vi "tpg361_ERR.vi"() -> ()   [LabVIEW 2019]
panel:
  out "Error Status":string
  out "Overall Status":bool
  out "Acknowledgement Status":bool
  out "err_out":errorcluster
  out "tpg361_visa 2":refnum<visa-resource-name>
  in  "tpg361_b2r 2":u32
  in  "tpg361_delay 3":u32=500
  in  "tpg361_delay 2":u32=500
  in  "tpg361_b2r":u32
  in  "err_in":errorcluster
  in  "tpg361_delay":u32=500
  in  "tpg361_visa":refnum<visa-resource-name>
  # "VISA"
  # "ERROR STATUS:\n0000 = No Error\n1000 = ERROR (controller error (see display on front\npanel)\n0100 = NO HWR (no hardware) \n0010 = PAR (inadmissible parameter) \n0001 = SYN (Syntax error)"
  # "DELAY"
  # "BYTE AT PORT"
  # "STATUS"
  # "ERROR"
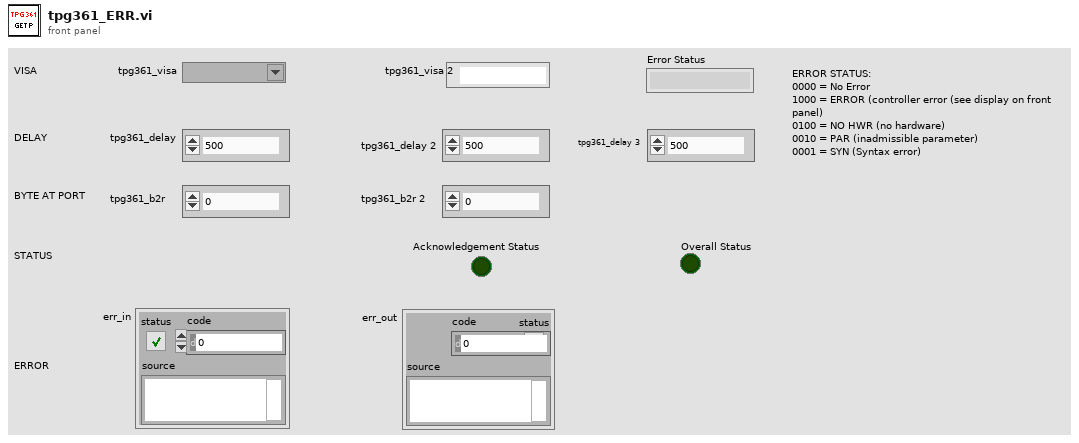
[diagram p1: front panel]
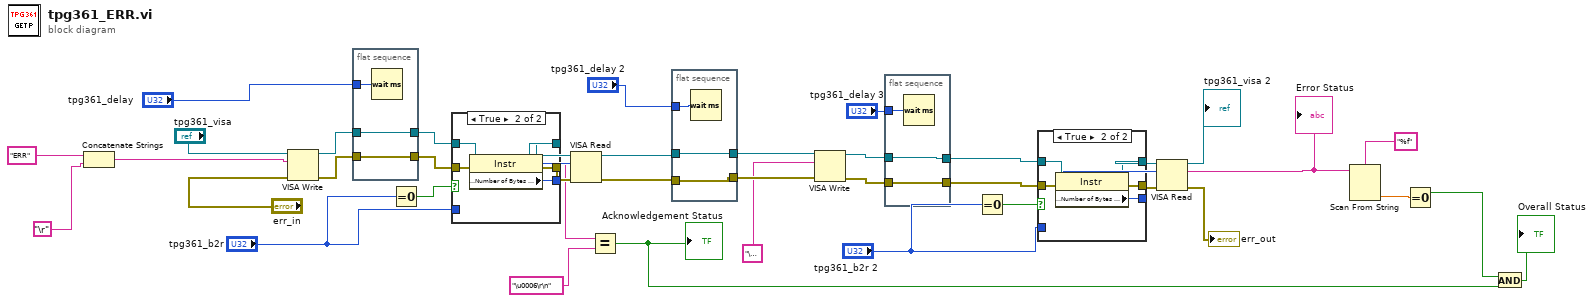
[diagram p0: block diagram]
diagram:
  n1 = Concatenate Strings("ERR" ("string"), "\r") -> (w13:string)
  n2 = VISA Write(VISA resource name="tpg361_visa", write buffer=w13, error in (no error)="err_in") -> (VISA resource name out=w39:refnum<visa-resource-name>, error out=w41:errorcluster)  [unwired: 1 out]
  n3 = flat-sequence {
    tunnel: w41 -> [w43]
    tunnel: [w43] -> w40
    tunnel: w39 -> [w42]
    tunnel: [w42] -> w38
    tunnel: "tpg361_delay" -> [w44]
    frame #0 {
      n4 = Wait (ms)(milliseconds to wait=w44) -> ()  [unwired: 1 out]
    }
  }
  n5 = Equal To 0?(x="tpg361_b2r") -> (x = 0?=w34:bool)
  n6 = case shown="True" w34 {
    tunnel: w40 -> [w46 w52]
    tunnel: w38 -> [w47 w51]
    tunnel: [w47 w50] -> w32
    tunnel: [w46 w49] -> w31
    tunnel: [w45 w48] -> w30
    tunnel: "tpg361_b2r" -> [w45 _]
    frame False {
    }
    frame True {
      n7 = property class="Instr"(reference=w51, error in=w52) -> (reference out=w50:refnum<visa-resource-name>, error out=w49:errorcluster, "Serial Settings:Number of Bytes at Serial Port"=w48:u32)
    }
  }
  n8 = VISA Read(VISA resource name=w32, byte count=w30, error in (no error)=w31) -> (VISA resource name out=w29:refnum<visa-resource-name>, read buffer=w10:string, error out=w28:errorcluster)  [unwired: 1 out]
  n9 = Equal?(x=w10, y="\u0006\r\n") -> (x = y?=w5:bool)
  "Acknowledgement Status" <- w5
  n10 = flat-sequence {
    tunnel: [w53] -> w26
    tunnel: w29 -> [w55]
    tunnel: [w55] -> w27
    tunnel: "tpg361_delay 2" -> [w54]
    tunnel: w28 -> [w53]
    frame #0 {
      n11 = Wait (ms)(milliseconds to wait=w54) -> ()  [unwired: 1 out]
    }
  }
  n12 = VISA Write(VISA resource name=w27, write buffer="\u0005", error in (no error)=w26) -> (VISA resource name out=w19:refnum<visa-resource-name>, error out=w18:errorcluster)  [unwired: 1 out]
  n13 = flat-sequence {
    tunnel: [w57] -> w25
    tunnel: [w58] -> w24
    tunnel: w19 -> [w58]
    tunnel: w18 -> [w57]
    tunnel: "tpg361_delay 3" -> [w56]
    frame #0 {
      n14 = Wait (ms)(milliseconds to wait=w56) -> ()  [unwired: 1 out]
    }
  }
  n15 = Equal To 0?(x="tpg361_b2r 2") -> (x = 0?=w23:bool)
  n16 = case shown="True" w23 {
    tunnel: w25 -> [w60 w66]
    tunnel: w24 -> [w61 w65]
    tunnel: [w61 w64] -> w22
    tunnel: [w60 w63] -> w21
    tunnel: [w59 w62] -> w20
    tunnel: "tpg361_b2r 2" -> [w59 _]
    frame False {
    }
    frame True {
      n17 = property class="Instr"(reference=w65, error in=w66) -> (reference out=w64:refnum<visa-resource-name>, error out=w63:errorcluster, "Serial Settings:Number of Bytes at Serial Port"=w62:u32)
    }
  }
  n18 = VISA Read(VISA resource name=w22, byte count=w20, error in (no error)=w21) -> (VISA resource name out=→"tpg361_visa 2":refnum<visa-resource-name>, read buffer=w3:string, error out=→"err_out":errorcluster)  [unwired: 1 out]
  "Error Status" <- w3
  n19 = Scan From String(format string="%f", input string=w3) -> (output 1=w1:dbl)  [unwired: 3 in, 3 out]
  n20 = Equal To 0?(x=w1) -> (x = 0?=w6:bool)
  n21 = And(x=w6, y=w5) -> (x .and. y?=→"Overall Status":bool)
